vi "DetermineNextPosition.vi"(1 "Nogo Positions":i32[](array[numeric])=[120, 240], 2 "GoTrial":bool=TRUE, 3 "Go Positions":i32[](array[numeric])=[0]) -> (0 "New Stage Position":i32)   [LabVIEW 2013]
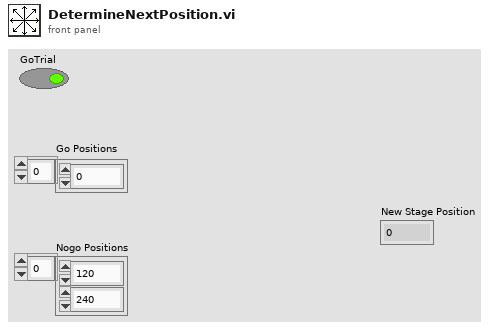
[diagram p1: front panel]
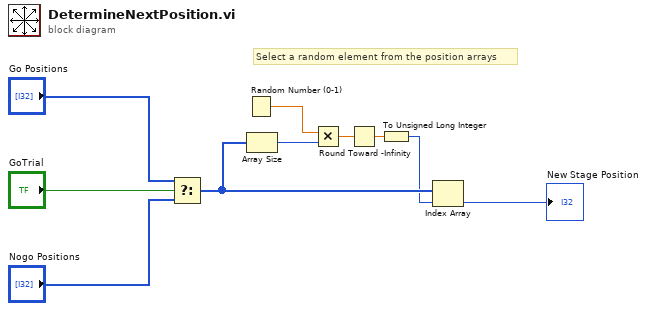
[diagram p0: block diagram]
diagram:
  # "Select a random element from the position arrays"
  n1 = Select(t="Go Positions", s="GoTrial", f="Nogo Positions") -> (s? t:f=w4:i32[])
  n2 = Random Number (0-1)() -> (number: 0 to 1=w6:dbl)
  n3 = Array Size(array=w4) -> (size(s)=w7:i32)
  n4 = Multiply(x=w6, y=w7) -> (x*y=w5:dbl)
  n5 = Round Toward -Infinity(1:w5) -> (0:w3:dbl)
  n6 = To Unsigned Long Integer(number=w3) -> (unsigned 32bit integer=w2:u32)
  n7 = Index Array(array=w4, index=w2) -> (element=→"New Stage Position":i32)
